vi "COMI DO Put All.vi"(10 "dwStatuses":u32, 11 "hDevice":u32) -> (2 "function return":i32, 3 "hDevice out":u32)   [LabVIEW 2017, in "Comidll.lvlib"]
doc: "int (COMI_DO_PutAll) (HANDLE hDevice, unsigned long dwStatuses);"
uses:
  <userlib>/Comidll/Comidll.lvlib
  <userlib>/Comidll/Comidll.dll
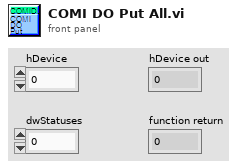
[diagram p1: front panel]
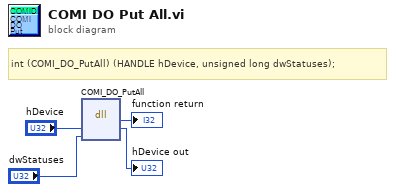
[diagram p0: block diagram]
diagram:
  # "int\t(COMI_DO_PutAll) (HANDLE hDevice, unsigned long dwStatuses);"
  n1 = dll-call lib="C:/Program Files/National Instruments/LabVIEW 2017/user.lib/Comidll/Comidll.*" fn="COMI_DO_PutAll"("hDevice"="hDevice", "dwStatuses"="dwStatuses") -> (→"function return":i32, "hDevice"=→"hDevice out":u32)  [unwired: 4 in, 2 out]
